vi "Read CSM-VIs.vi"(6 "Config Path":path, 8 "Error In":errorcluster caption="Error in (no error)") -> (0 "Error Out":errorcluster, 3 "Array":string[](array[string]))   [LabVIEW 2017, in "CSM-Helper API with lvcsm Support.lvlib"]
uses:
  CSM-Helper API with lvcsm Support.lvlib
  <vilib>/Utility/config.llb/NI_LVConfig.lvlib
  lvcsmFile/lvcsm File Support.lvlib
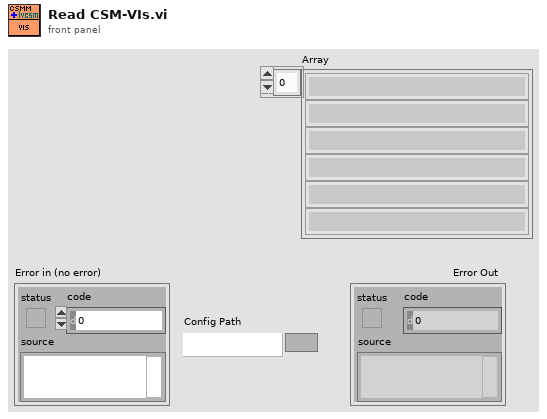
[diagram p1: front panel]
types:
  T1 = typedef "NI_LVConfig.lvlib/Config Data RefNum.ctl" = refnum<k1>
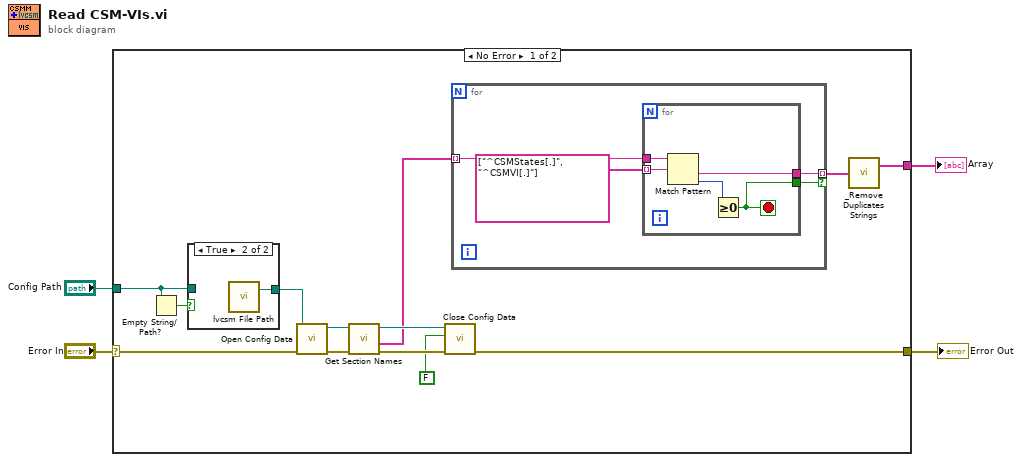
[diagram p0: block diagram]
diagram:
  n1 = case shown="No Error" "Error In" {
    selector: "Error In" -> [w15 w29]
    tunnel: [w16 w29] -> w3
    tunnel: "Config Path" -> [w17 _]
    tunnel: [w5 _] -> w1
    frame No Error {
      n2 = Empty String/Path?(string/path=w17) -> (empty?=w13:bool)
      n3 = case shown="True" w13 {
        tunnel: [w27 w28] -> w12
        tunnel: w17 -> [w27 _]
        frame False {
        }
        frame True {
          n4 = call "lvcsm File Path.vi"() -> ("Appended Path"=w28:path)  [unwired: 3 in]
        }
      }
      n5 = call <vilib>:"Open Config Data.vi"("error in (no error)"=w15, "configuration file path"=w12) -> ("error out"=w8:errorcluster, "refnum"=w14:T1)  [unwired: 7 in, 1 out]
      n6 = call <vilib>:"Get Section Names.vi"("error in (no error)"=w8, "refnum"=w14) -> ("error out"=w11:errorcluster, "section names"=w7:string[], "refnum out"=w10:T1)  [unwired: 7 in]
      n7 = call <vilib>:"Close Config Data.vi"("error in (no error)"=w11, "write file if changed (T)"=FALSE, "refnum"=w10) -> ("error out"=w16:errorcluster)  [unwired: 7 in, 1 out]
      n8 = for {
        tunnel: w7 -> [w21] mode=indexing
        tunnel: [w19] -> w6 mode=indexing if=w18
        n9 = for {
          tunnel: w21 -> [w26]
          tunnel: string[] ["^CSMStates[.]", "^CSMVI[.]"] ("regular expression") -> [w25] mode=indexing
          tunnel: [w23] -> w19
          tunnel: [w22] -> w18
          stop <- w22 stop-if-true
          n10 = Match Pattern(string=w26, regular expression=w25) -> (after substring=w23:string, offset past match=w24:i32)  [unwired: 1 in, 2 out]
          n11 = Greater Or Equal To 0?(x=w24) -> (x >= 0?=w22:bool)
        }
      }
      n12 = call "_Remove Duplicates Strings.vi"("Input Array"=w6) -> ("Output Array"=w5:string[])  [unwired: 1 out]
    }
    frame Error {
    }
  }
  "Error Out" <- w3
  "Array" <- w1
